vi "(RAG) Load PDF into KB.vi"(0 "Python Session Refnum in":refnum<k35>, 1 "Chroma Database Folder":path, 2 "Knowledge Base Name":string, 3 "Clear DB?":bool=TRUE, 5 "PDF Folder to Build KB":path, 7 "Chunk Settings":T1={"Chunk Size"=1000, "Chunk Overlap"=100}, 9 "Separators":string="\"\\n\"", 11 "error in":errorcluster, 12 "Embedding Model Base URL":string, 13 "Embedding Model":string) -> (4 "Python Session Refnum out":refnum<k35>, 8 "Log":string, 15 "error out":errorcluster)   [LabVIEW 2023, in "LabVIEW RAG.lvlib"]
uses:
  LabVIEW RAG.lvlib
  Typedefs/RAG Chunk Settings.ctl
  AI RAG Globals.vi
  labview-ai-share/LabVIEW AI Base.lvlib
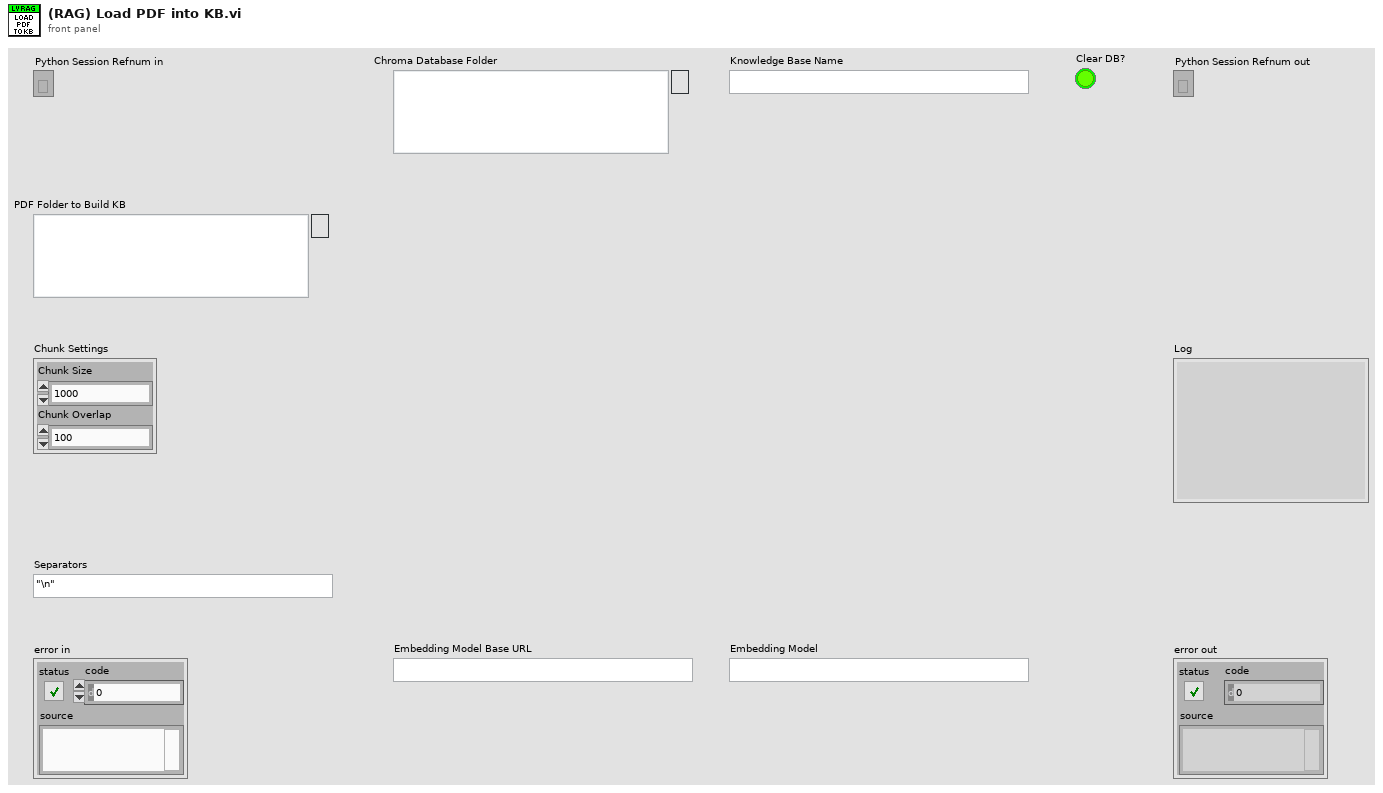
[diagram p1: front panel]
types:
  T1 = typedef "LabVIEW RAG.lvlib/RAG Chunk Settings.ctl" = cluster{"Chunk Size":u32, "Chunk Overlap":u32}
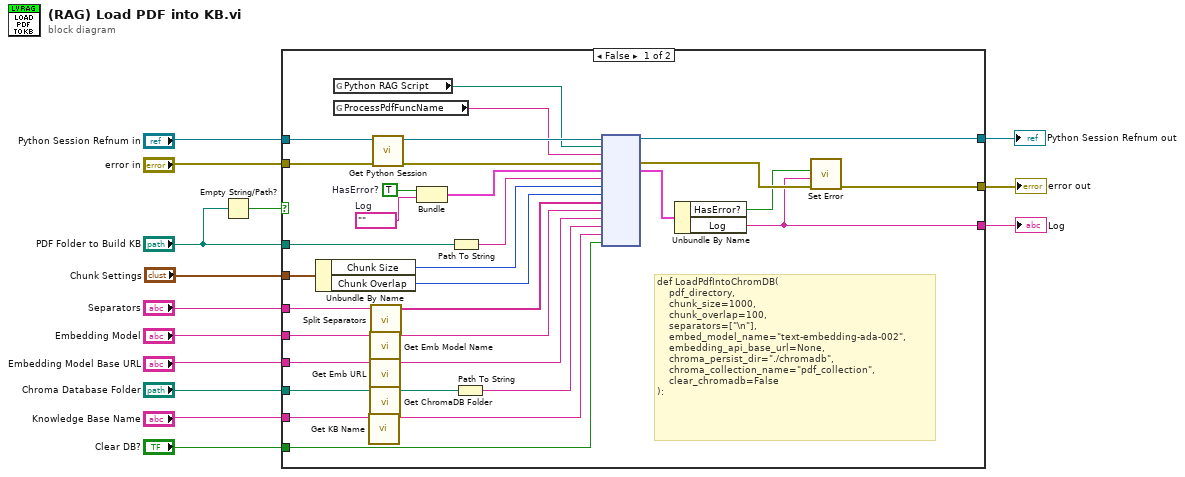
[diagram p0: block diagram]
diagram:
  n1 = Empty String/Path?(string/path="PDF Folder to Build KB") -> (empty?=w2:bool)
  n2 = case shown="False" w2 {
    tunnel: "Knowledge Base Name" -> [w45 _]
    tunnel: "Embedding Model Base URL" -> [w44 _]
    tunnel: "Embedding Model" -> [w43 _]
    tunnel: "Chroma Database Folder" -> [w42 _]
    tunnel: [w40 w47] -> w10
    tunnel: "PDF Folder to Build KB" -> [w39 _]
    tunnel: "error in" -> [w37 w46]
    tunnel: "Python Session Refnum in" -> [w36 w47]
    tunnel: "Separators" -> [w31 _]
    tunnel: "Clear DB?" -> [w26 _]
    tunnel: [w21 w46] -> w5
    tunnel: [w19 _] -> w4
    tunnel: "Chunk Settings" -> [w18 _]
    frame False {
      w24 = ""  # Log
      w25 = TRUE  # HasError?
      # "def LoadPdfIntoChromDB(\n    pdf_directory,\n    chunk_size=1000,\n    chunk_overlap=100,\n    separators=[\"\\n\"],\n    embed_model_name=\"text-embedding-ada-002\",\n    embedding_api_base_url=None,\n    chroma_persist_dir=\"./chromadb\",\n    chroma_collection_name=\"pdf_collection\",\n    clear_chromadb=False\n):"
      n3 = Unbundle By Name(w18) -> ("Chunk Size"=w17:u32, "Chunk Overlap"=w16:u32)
      n4 = global read "AI RAG Globals.vi" "Python RAG Script"() -> (w32:path)
      n5 = global read "AI RAG Globals.vi" "ProcessPdfFuncName"() -> (w33:string)
      n6 = call "Get KB Name.vi"("KB Name"=w45) -> ("KB Name"=w27:string)  [unwired: 10 in]
      n7 = call "Get Emb Model Name.vi"("Embedding Model Name in"=w43) -> ("Embedding Model Name out"=w30:string)  [unwired: 10 in]
      n8 = call "Get Emb URL.vi"("Embedding Model URL in"=w44) -> ("Embedding Model URL out"=w29:string)  [unwired: 10 in]
      n9 = call "Get ChromaDB Folder.vi"("ChromaDB Folder in"=w42) -> ("ChromaDB Folder out"=w34:path)  [unwired: 10 in]
      n10 = call "Split Separators.vi"("Separators"=w31) -> ("Separator List"=w15:string[])  [unwired: 10 in]
      n11 = call "Get Python Session.vi"("Python Session in"=w36) -> ("Python Session out"=w35:refnum<k35>)  [unwired: 10 in]
      n12 = Bundle("HasError?"=w25, "Log"=w24) -> (w23:cluster{"HasError?":bool, "Log":string})  [unwired: 1 in]
      n13 = Path To String(path=w39) -> (string=w41:string)
      n14 = Path To String(path=w34) -> (string=w28:string)
      n15 = node(w35, w32, w33, w37, w23, w41, w17, w16, w15, w30, w29, w28, w27, w26) -> (w40:refnum<k35>, w38:errorcluster, w22:cluster{"HasError?":bool, "Log":string})  [unwired: 9 in, 2 out]
      n16 = Unbundle By Name(w22) -> ("HasError?"=w20:bool, "Log"=w19:string)
      n17 = call "Set Error.vi"("error in"=w38, "Log"=w19, "HasError?"=w20) -> ("error out"=w21:errorcluster)  [unwired: 8 in]
    }
    frame True {
    }
  }
  "Python Session Refnum out" <- w10
  "error out" <- w5
  "Log" <- w4
